vi "LSX Get RFID.vi"(7 "plRFID":i32, 8 "error in (no error)":errorcluster, 9 "bank":i32, 10 "slot":i32, 11 "lLSID":i32) -> (0 "error out":errorcluster, 3 "function return":i32, 5 "plRFID out":i32)   [LabVIEW 2016, in "Tango_DLL.lvlib"]
doc: "TANGOAPI int TANGOCALL LSX_GetRFID (int lLSID, int slot, int bank, int *plRFID);"
uses:
  Tango_DLL.lvlib
  2017/Microscope Control/Device Library/Stages/Marzhauser/SCAN IM 120 x 80/Tango DLL VIs/Tango_DLL.dll
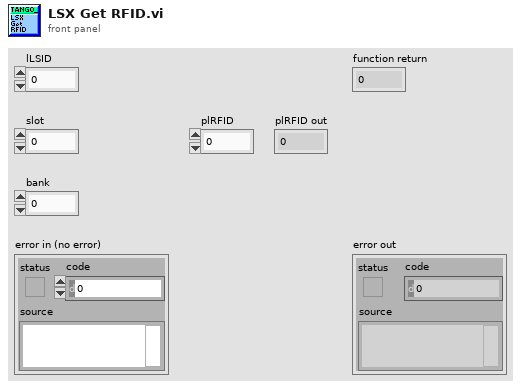
[diagram p1: front panel]
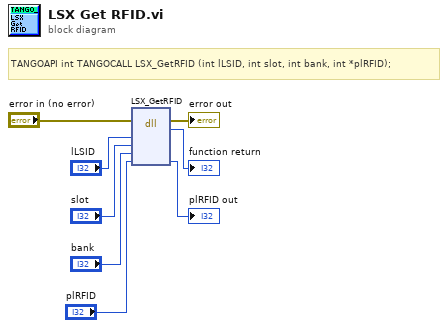
[diagram p0: block diagram]
diagram:
  # "TANGOAPI int TANGOCALL LSX_GetRFID (int lLSID, int slot, int bank, int *plRFID);"
  n1 = dll-call lib="C:/Users/4PiSMS/Documents/Microscope Control/2017/Microscope Control/Device Library/Stages/Marzhauser/SCAN IM 120 x 80/Tango DLL VIs/Tango_DLL.*" fn="LSX_GetRFID"(error in="error in (no error)", "lLSID"="lLSID", "slot"="slot", "bank"="bank", "plRFID"="plRFID") -> (error out=→"error out":errorcluster, →"function return":i32, "plRFID"=→"plRFID out":i32)  [unwired: 5 in, 1 out]
